vi "Sinusoidal Force.vi"(6 "Cycle Count (0)":i32, 7 "Period":dbl=0.2 min=0.2 max=429496729.5 step=0.1 format="%#.1f", 8 "error in (no error)":errorcluster, 9 "Device and Axis":string, 10 "Force Amplitude":i32 min=-700 max=700, 11 "VISA resource name":refnum<visa-resource-name>) -> (0 "error out":errorcluster, 3 "VISA resource name out":refnum<visa-resource-name>)   [LabVIEW 2018, in "Zaber A Series.lvlib"]
doc: "Set the sinusoidal force output on Zaber devices that support force output mode, such as the X-DMQ-DE. Sinusoidal force can be added to continuous force created with the Force VI.\n\nThe input force amplitude value is a peak (not peak-to-peak) quantity in a unitless device-specific force resolution ; consult your device manual for the conversion from standard force units. \n\nThe period input is the time for a full sinusoid in milliseconds, with a resolution of 0.1ms.\n\nThe optional cycle count input specified how many cycles of output to produce. If zero, the output will oscillate until stopped.\n\nSetting the amplitude input to zero will end the oscillation at the next cycle boundary. To stop force output immediately use the Force Off VI.\n\nThis VI requires that the VISA serial port input has already been configured and opened."
uses:
  Zaber A Series.lvlib
  Private/All Commands.ctl
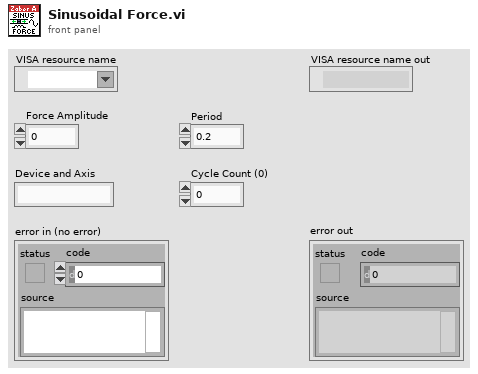
[diagram p1: front panel]
types:
  T1 = typedef "Zaber A Series.lvlib/All Commands.ctl" = string
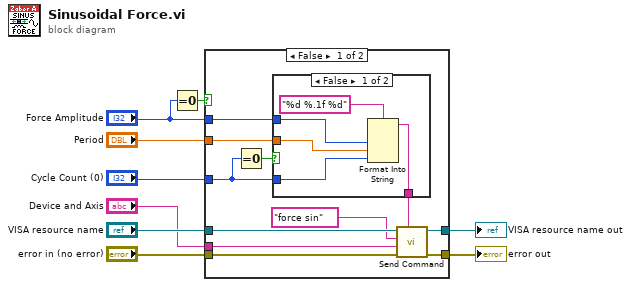
[diagram p0: block diagram]
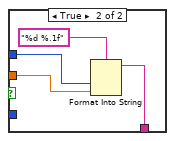
[diagram p2: hidden frame]
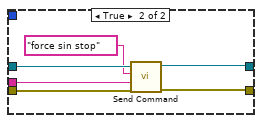
[diagram p3: hidden frame]
diagram:
  n1 = Equal To 0?(x="Force Amplitude") -> (x = 0?=w3:bool)
  n2 = case shown="False" w3 {
    tunnel: "VISA resource name" -> [w20 w35]
    tunnel: [w19 w33] -> w8
    tunnel: "error in (no error)" -> [w18 w34]
    tunnel: [w17 w32] -> w6
    tunnel: "Device and Axis" -> [w16 w31]
    tunnel: "Force Amplitude" -> [w12 _]
    tunnel: "Period" -> [w15 _]
    tunnel: "Cycle Count (0)" -> [w13 _]
    frame False {
      n3 = Equal To 0?(x=w13) -> (x = 0?=w14:bool)
      n4 = case shown="False" w14 {
        tunnel: w12 -> [w24 w27]
        tunnel: w15 -> [w23 w26]
        tunnel: w13 -> [w22 _]
        tunnel: [w21 w28] -> w11
        frame False {
          n5 = Format Into String(format string="%d %.1f %d", w24, w23, w22) -> (resulting string=w21:string)  [unwired: 2 in, 1 out]
        }
        frame True {
          n6 = Format Into String(format string="%d %.1f", w27, w26) -> (resulting string=w28:string)  [unwired: 2 in, 1 out]
        }
      }
      n7 = call "Send Command.vi"("Data"=w11, "error in (no error)"=w18, "Device and Axis"=w16, "Command"=T1 "force sin" ("Complete Command List"), "VISA resource name"=w20) -> ("error out"=w17:errorcluster, "VISA resource name out"=w19:refnum<visa-resource-name>)  [unwired: 1 in, 4 out]
    }
    frame True {
      n8 = call "Send Command.vi"("error in (no error)"=w34, "Device and Axis"=w31, "Command"=T1 "force sin stop" ("Complete Command List"), "VISA resource name"=w35) -> ("error out"=w32:errorcluster, "VISA resource name out"=w33:refnum<visa-resource-name>)  [unwired: 2 in, 4 out]
    }
  }
  "VISA resource name out" <- w8
  "error out" <- w6
